vi "Set Equation Para.vi"(8 "error in (no error)":errorcluster, 10 "parameter":variant, 11 "PDE_2ndOrder_ConstPara in":refnum<class "NI_PDE_2ndOrder_ConstPara.lvclass">) -> (0 "error out":errorcluster, 3 "PDE_2ndOrder_ConstPara out":refnum<class "NI_PDE_2ndOrder_ConstPara.lvclass">)   [LabVIEW 2020, in "NI_PDE.lvlib" / "NI_PDE_2ndOrder_ConstPara.lvclass"]
uses:
  <vilib>/gmath/pde.llb/PDEClass/PDE_2ndOrder_ConstPara/NI_PDE_2ndOrder_ConstPara.lvclass
  <vilib>/gmath/pde.llb/PDEClass/PDE_2ndOrder_ConstPara/Para Data.ctl
  <vilib>/gmath/pde.llb/PDEClass/PDE_2ndOrder_ConstPara/NI_PDE_2ndOrder_ConstPara.lvclass/NI_PDE_2ndOrder_ConstPara.ctl
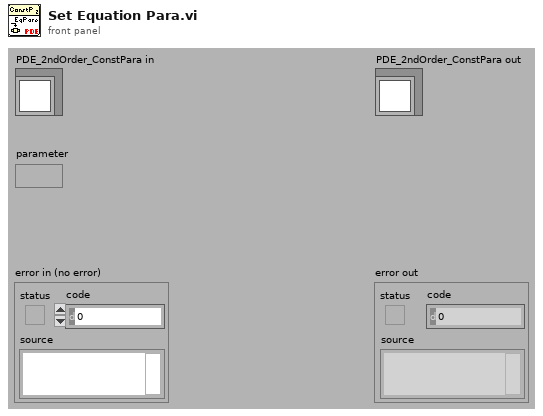
[diagram p1: front panel]
types:
  T1 = typedef "NI_PDE.lvlib/NI_PDE_2ndOrder_ConstPara.lvclass/Para Data.ctl" = cluster{"k":dbl, "a":dbl}
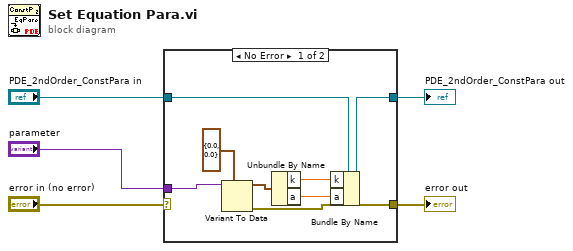
[diagram p0: block diagram]
diagram:
  n1 = case shown="No Error" "error in (no error)" {
    selector: "error in (no error)" -> [_ w15]
    tunnel: "PDE_2ndOrder_ConstPara in" -> [w10 w14]
    tunnel: [w9 w14] -> w4
    tunnel: [w8 w15] -> w3
    tunnel: "parameter" -> [w12 _]
    frame No Error {
      n2 = Variant To Data(type=T1 {"k"=0.0, "a"=0.0} ("para data"), Variant=w12) -> (data=w11:T1, error out=w8:errorcluster)  [unwired: 1 in]
      n3 = Unbundle By Name(w11) -> ("k"=w7:dbl, "a"=w6:dbl)
      n4 = Bundle By Name(cluster=w10, "k"=w7, "a"=w6) -> (w9:refnum<class "NI_PDE_2ndOrder_ConstPara.lvclass">)
    }
    frame Error {
    }
  }
  "PDE_2ndOrder_ConstPara out" <- w4
  "error out" <- w3
